vi "Write Message Flattener.vi"(10 "Message Flattener.lvclass":refnum<class "Message Flattener.lvclass">, 11 "Message Stream in":refnum<class "Message Stream.lvclass">) -> (3 "Message Stream out":refnum<class "Message Stream.lvclass">)   [LabVIEW 2020, in "Message Stream.lvclass"]
uses:
  Message Stream.lvclass
  Message Flattener/Message Flattener.lvclass
  Message Stream.lvclass/Message Stream.ctl
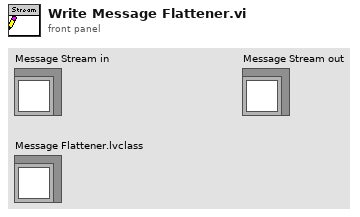
[diagram p1: front panel]
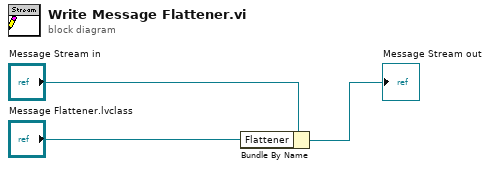
[diagram p0: block diagram]
diagram:
  n1 = Bundle By Name(cluster="Message Stream in", "Flattener"="Message Flattener.lvclass") -> (→"Message Stream out":refnum<class "Message Stream.lvclass">)
